vi "serialwritefpga.vi"(0 "FPGA VI Reference In":refnum<k20>, 1 "Port":T1(ring)=enum."1", 2 "String":string, 3 "error in":errorcluster caption="error out") -> (5 "FPGA VI Reference Out":refnum<k20>, 6 "error out":errorcluster)   [LabVIEW 2010]
uses:
  <vilib>/rvi/interface/nirviMethod/nirviMethod.xnode
  C:/Users/HAGAR-IV/Desktop/Zeugs/markus/version feb 2012/test/Auslesenkopiekopie2.vi
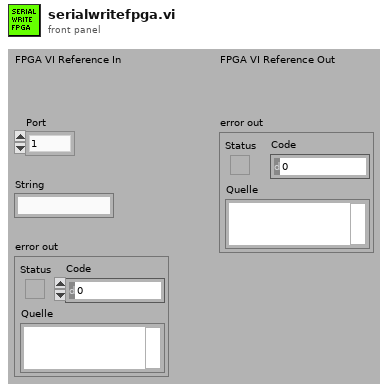
[diagram p1: front panel]
types:
  T1 = enum8{"0", "1", "2", "3", "4", "5", "6", "7", "8"}
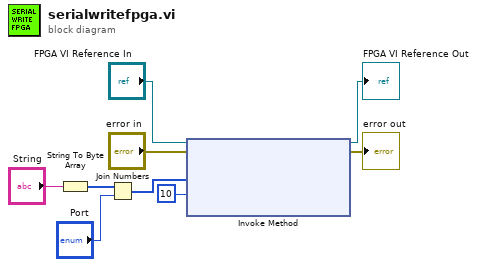
[diagram p0: block diagram]
diagram:
  n1 = String To Byte Array(string="String") -> (unsigned byte array=w2:u8[])
  n2 = Join Numbers(hi=w2, lo="Port") -> ((hi.lo)=w3:u16[])
  n3 = xnode "Invoke Method"("FPGA VI Reference In"="FPGA VI Reference In", "error in"="error in", "Data"=w3, "Timeout (ms)"=10) -> ("FPGA VI Reference Out"=→"FPGA VI Reference Out":refnum<k20>, "error out"=→"error out":errorcluster)  [unwired: 1 out]
